vi "Request Header Analysis.vi"(11 "请求首部字段":string) -> (2 "value":string[](array[string]), 3 "key":string[](array[string]))   [LabVIEW 2019, in "HTTP Server.lvlib"]
uses:
  HTTP Server.lvlib
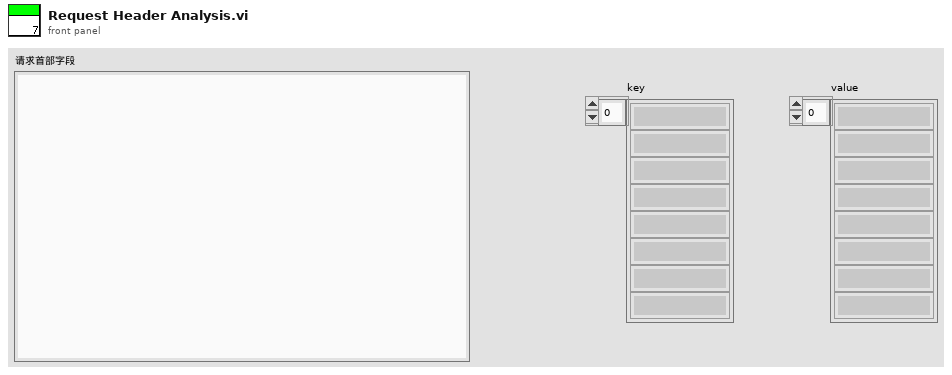
[diagram p1: front panel]
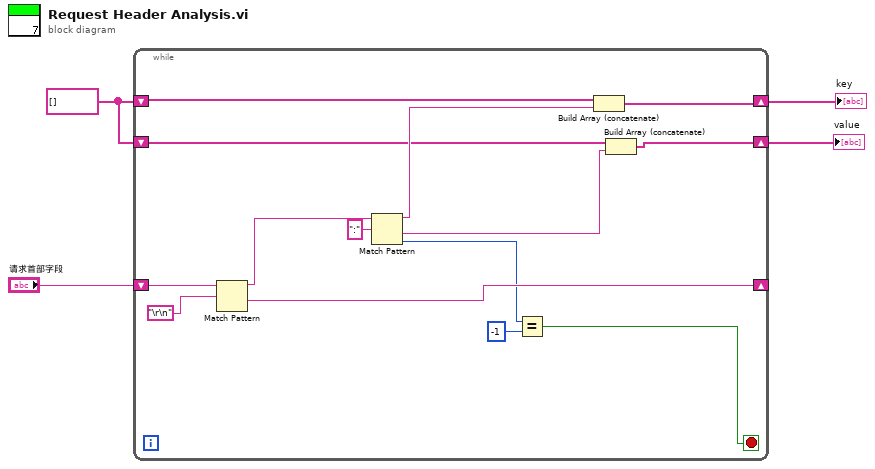
[diagram p0: block diagram]
diagram:
  w3 = string[] []
  n1 = while {
    shift-right: [w16] -> _
    shift-left: "请求首部字段" -> [w18]
    shift-right: [w11] -> w2
    shift-left: w3 -> [w13]
    shift-right: [w9] -> w1
    shift-left: w3 -> [w10]
    stop <- w5 stop-if-true
    n2 = Match Pattern(string=w18, regular expression="\r\n") -> (before substring=w15:string, after substring=w16:string)  [unwired: 1 in, 2 out]
    n3 = Match Pattern(string=w15, regular expression=":" ("正则表达式")) -> (before substring=w12:string, after substring=w8:string, offset past match=w7:i32)  [unwired: 1 in, 1 out]
    n4 = Equal?(x=w7, y=-1) -> (x = y?=w5:bool)
    n5 = Build Array (concatenate)(w13, w12) -> (w11:string[])
    n6 = Build Array (concatenate)(w10, w8) -> (w9:string[])
  }
  "key" <- w2
  "value" <- w1
